vi "Flush TCP Buffer.vi"(8 "error in (no error)":errorcluster, 11 "TCP Network Connection in":refnum<k5>) -> (0 "error out":errorcluster, 3 "TCP Network Connection out":refnum<k5>)   [LabVIEW 2024, in "OptoMMP.lvlib"]
doc: "Clears the TCP buffer by reading a large amount of bytes. If a TCP read timeout occurs, this indicates the TCP buffer is empty and the resulting error is then cleared to allow subsequent blocks to execute.\n\nLast updated: 7/31/2025"
uses:
  <vilib>/ErrorRing/Error Ring.xnode
  <instrlib>/OptoMMP/OptoMMP.lvlib
panel:
  # "Copyright (c) 2025 California Institute of Technology (Caltech).\nU.S. Government sponsorship acknowledged.\n\nLicensed under the Apache License, Version 2.0 (the \"License\");\nyou may not use this file except in compliance with the License.\nYou may obtain a copy of the License at\n\n    http://www.apache.org/licenses/LICENSE-2.0\n\nUnless required by applicable law or agreed to in writing, software\ndistributed under the License is distributed on an \"AS IS\" BASIS,\nWITHOUT WARRANTIES OR CONDITIONS OF ANY KIND, either express or implied.\nSee the License for the specific language governing permissions and\nlimitations under the License."
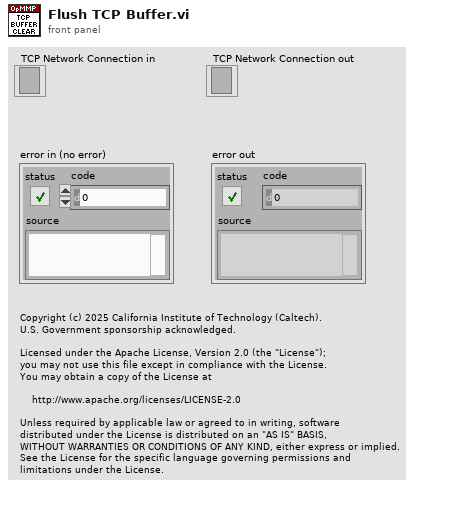
[diagram p1: front panel]
types:
  T1 = enum16{"Standard", "Buffered", "CRLF", "Immediate"}
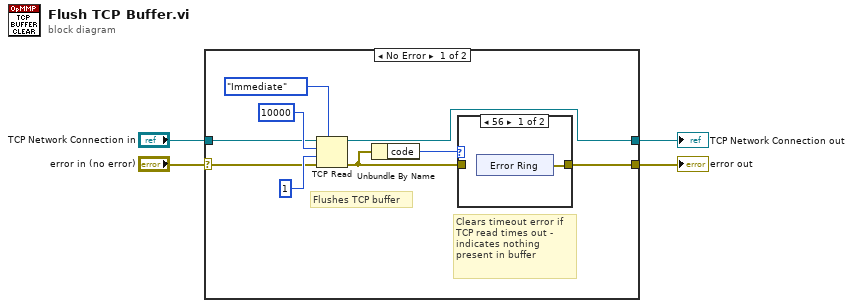
[diagram p0: block diagram]
diagram:
  n1 = case shown="No Error" "error in (no error)" {
    selector: "error in (no error)" -> [w5 w18]
    tunnel: [w13 w17] -> w4
    tunnel: [w8 w18] -> w3
    tunnel: "TCP Network Connection in" -> [w6 w17]
    frame No Error {
      # "Clears timeout error if \nTCP read times out - indicates nothing present in buffer"
      # "Flushes TCP buffer"
      n2 = TCP Read(connection ID=w6, bytes to read=10000, error in (no error)=w5, 7:T1."Immediate" ("mode (standard)"), 9:1 ("timeout ms (25000)")) -> (connection ID out=w13:refnum<k5>, error out=w9:errorcluster)  [unwired: 1 out]
      n3 = Unbundle By Name(w9) -> ("code"=w7:i32)
      n4 = case shown="56" w7 {
        tunnel: [w14 w16] -> w8
        tunnel: w9 -> [_ w16]
        frame 56 {
          n5 = xnode "Error Ring"() -> ("error out"=w14:errorcluster)
        }
        frame 0, Default {
        }
      }
    }
    frame Error {
    }
  }
  "TCP Network Connection out" <- w4
  "error out" <- w3
